vi "Init Server.vi"(6 "ms timeout listening":i32=50, 7 "ms create listener":i32=3000, 8 "error in (no error)":errorcluster, 9 "ms send status":i32=1000, 10 "ms rec message":i32=500, 11 "Server in":refnum<class "TCP-Server.lvclass">) -> (0 "error out":errorcluster, 3 "Server out":refnum<class "TCP-Server.lvclass">)   [LabVIEW 2018, in "TCP-Server.lvclass"]
uses:
  TCP-Server.lvclass
  TCP-Server.lvclass/TCP-Server.ctl
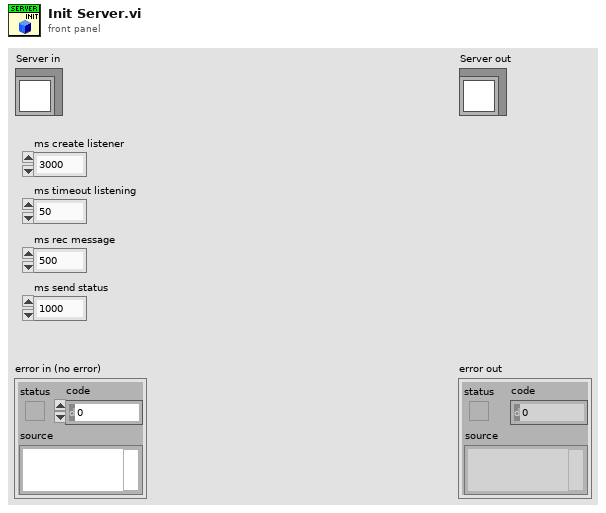
[diagram p1: front panel]
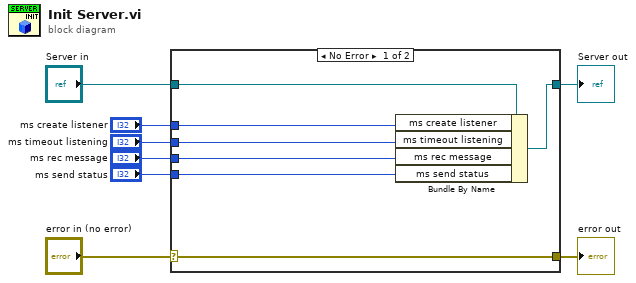
[diagram p0: block diagram]
diagram:
  n1 = case shown="No Error" "error in (no error)" {
    selector: "error in (no error)" -> [w15 w16]
    tunnel: [w15 w16] -> w7
    tunnel: [w13 w17] -> w5
    tunnel: "Server in" -> [w14 w17]
    tunnel: "ms send status" -> [w12 _]
    tunnel: "ms rec message" -> [w11 _]
    tunnel: "ms timeout listening" -> [w10 _]
    tunnel: "ms create listener" -> [w9 _]
    frame No Error {
      n2 = Bundle By Name(cluster=w14, "ms create listener"=w9, "ms timeout listening"=w10, "ms rec message"=w11, "ms send status"=w12) -> (w13:refnum<class "TCP-Server.lvclass">)
    }
    frame Error {
    }
  }
  "error out" <- w7
  "Server out" <- w5
